vi "Display stack trace log global.vi"(3 "return code":u8) -> ()   [LabVIEW 2018, in "LV-0mq-Julia_roundtrip-lib.lvlib"]
uses:
  LV-0mq-Julia_roundtrip-lib.lvlib
  jl stack traces global.vi
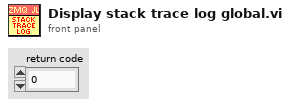
[diagram p1: front panel]
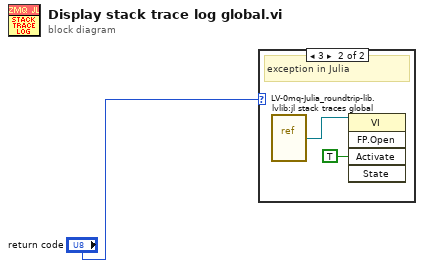
[diagram p0: block diagram]
diagram:
  n1 = case shown="3" "return code" {
    frame 0, Default {
    }
    frame 3 {
      # "exception in Julia"
      n2 = vi-ref "LV-0mq-Julia_roundtrip-lib.lvlib:jl stack traces global.vi"() -> (w2:refnum<vi>)
      n3 = invoke class="VI" method="FP.Open"(reference=w2, "Activate"=TRUE ("Activate?")) -> ()  [unwired: 3 in, 5 out]
    }
  }
